vi "Write CleanSession.vi"(8 "error in (no error)":errorcluster, 10 "CleanSession":bool, 11 "Session in":refnum<class "Session.lvclass">) -> (0 "error out":errorcluster, 3 "Session out":refnum<class "Session.lvclass">)   [LabVIEW 2013, in "MQTT Base.lvlib" / "Session.lvclass"]
uses:
  Session.lvclass
  Session.lvclass/Session.ctl
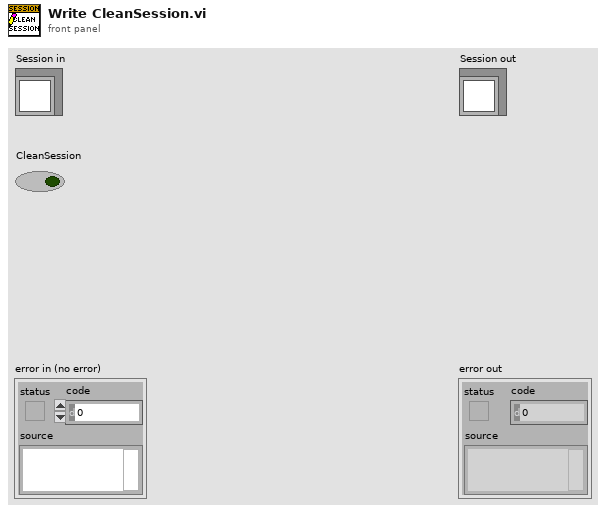
[diagram p1: front panel]
types:
  T1 = typedef "MQTT Base.lvlib/Session.lvclass/Session State -- cluster.ctl" = cluster{"CleanSession":bool, "Client ID":string, "Subscriptions":T2[], "Pending Transmissions":T4[], "Pending ACKs":T5[]}
  T2 = typedef "MQTT_Control_Packets.lvlib/SUBSCRIBE.lvclass/Topic Subscription -- cluster.ctl" = cluster{"Topic Filter":string, "QoS":T3}
  T3 = typedef "MQTT_Control_Packets.lvlib/ControlPacket.lvclass/QualityOfService -- enum.ctl" = enum16{"0 (At Most Once)", "1 (At Least Once)", "2 (Exactly Once)"}
  T4 = typedef "MQTT_Control_Packets.lvlib/ControlPacket.lvclass/Pending Transmission -- cluster.ctl" = cluster{"Message":refnum<class "ControlPacket.lvclass">, "QoS":T3, "Tx-Rx":bool}
  T5 = typedef "MQTT Base.lvlib/Session.lvclass/Pending ACKs -- cluster.ctl" = cluster{"Message":refnum<class "ControlPacket.lvclass">, "[ACK]":refnum<notifier>[], "Packet Identifier":u16}
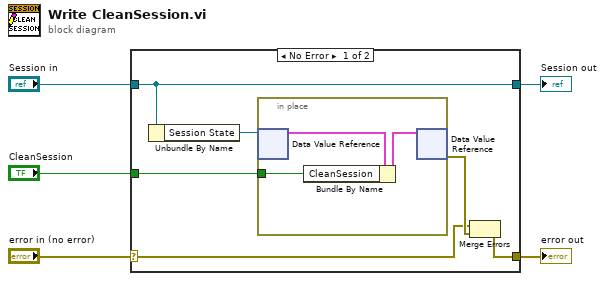
[diagram p0: block diagram]
diagram:
  n1 = case shown="No Error" "error in (no error)" {
    selector: "error in (no error)" -> [w7 w15]
    tunnel: [w6 w15] -> w4
    tunnel: [w11 w16] -> w2
    tunnel: "Session in" -> [w11 w16]
    tunnel: "CleanSession" -> [w9 _]
    frame No Error {
      n2 = Unbundle By Name(w11) -> ("Session State"=w10:refnum<data-value>)
      n3 = in-place {
        in-place-border: w9 -> [w12]
        n4 = in-place-dvr #1(w10) -> (w14:T1)  [unwired: 1 out]
        n5 = Bundle By Name(cluster=w14, "CleanSession"=w12) -> (w13:T1)
        n6 = in-place-dvr #1(w13) -> (w8:errorcluster)  [unwired: 1 out]
      }
      n7 = Merge Errors(w7, w8) -> (w6:errorcluster)
    }
    frame Error {
    }
  }
  "error out" <- w4
  "Session out" <- w2
